vi "Sub UI Update i box.vi"(8 "error in (no error)":errorcluster, 11 "LF2R IDE in":refnum<class "LF2R IDE.lvclass">) -> (0 "error out":errorcluster, 3 "LF2R IDE out":refnum<class "LF2R IDE.lvclass">)   [LabVIEW 2018, in "LF2R IDE.lvlib" / "LF2R IDE.lvclass"]
uses:
  LF2R IDE.lvclass
  LF2R IDE.lvclass/LF2R IDE.ctl
  Image/Image Process.lvclass
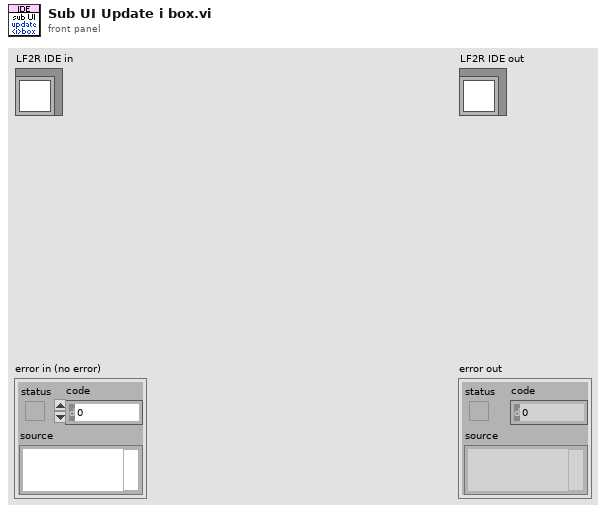
[diagram p1: front panel]
types:
  T1 = typedef "IMAQ Image.ctl" = refnum<image>
  T2 = typedef "Data Parser.lvclass/frame i data.ctl" = cluster{"kind":string, "x":string, "y":string, "w":string, "h":string, "dvx":string, "dvy":string, "dvz":string, "fall":string, "arest":string, "vrest":string, "bdefend":string, "injury":string, "zwidth":string, "effect":string, "catchingact":string, "caughtact":string}
  T3 = cluster{"Fill Color":u32, "Border Color":u32, "Show?":bool}
  T4 = cluster{"x":string, "y":string, "w":string, "h":string}
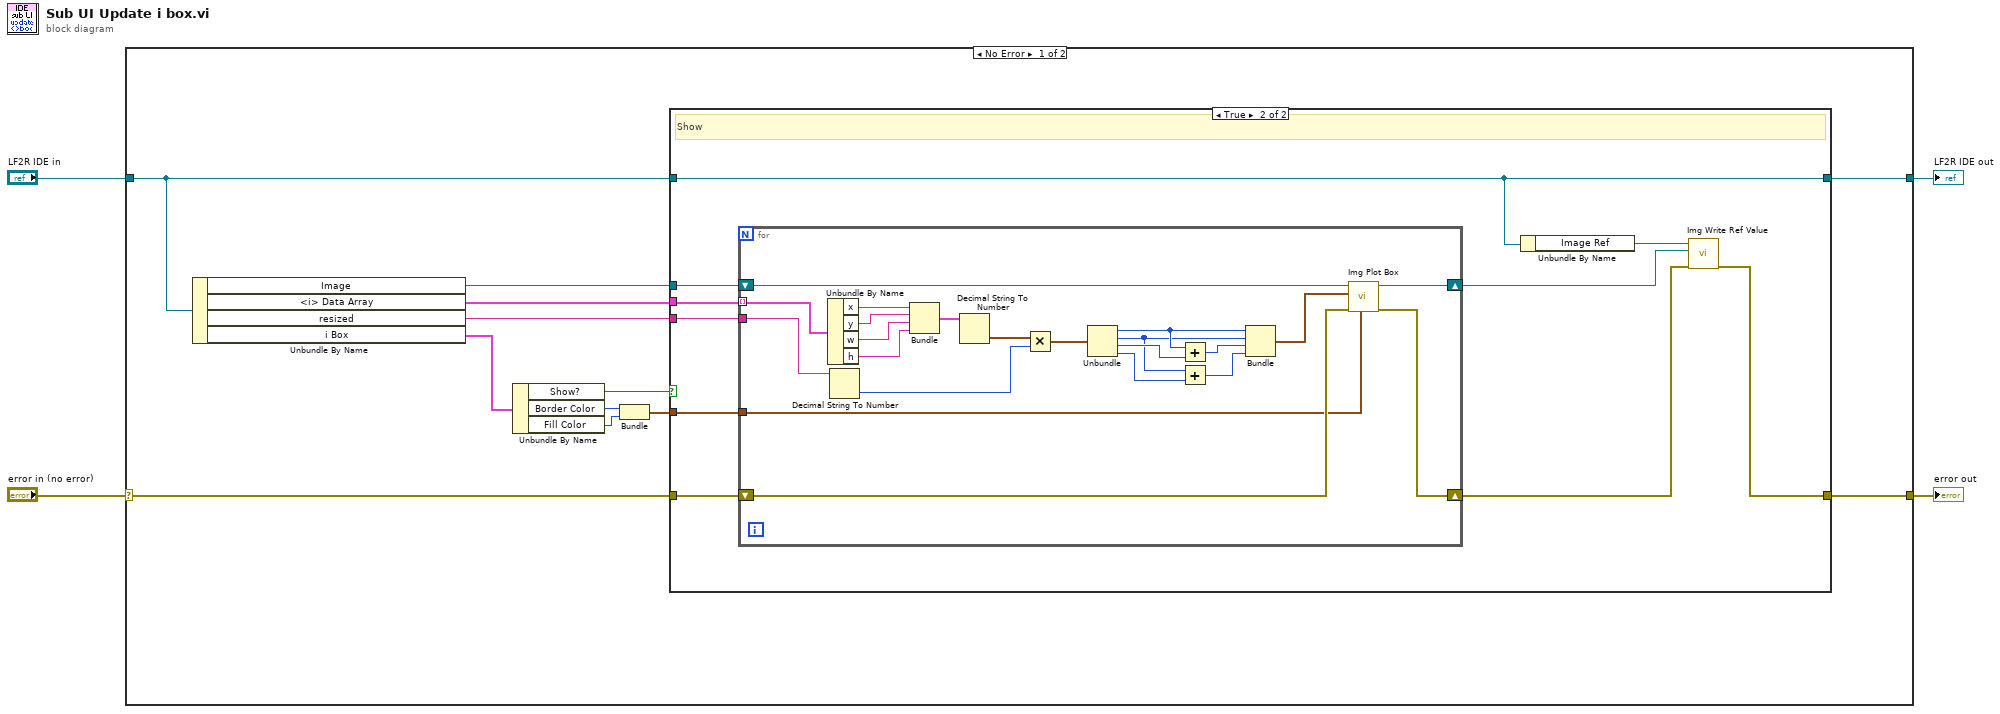
[diagram p0: block diagram]
diagram:
  n1 = case shown="No Error" "error in (no error)" {
    selector: "error in (no error)" -> [w14 w52]
    tunnel: [w12 w52] -> w3
    tunnel: [w9 w51] -> w1
    tunnel: "LF2R IDE in" -> [w13 w51]
    frame No Error {
      n2 = Unbundle By Name(w13) -> ("Image"=w16:T1, "<i> Data Array"=w15:T2[], "resized"=w11:string, "i Box"=w10:T3)
      n3 = Unbundle By Name(w10) -> ("Show?"=w8:bool, "Border Color"=w7:u32, "Fill Color"=w6:u32)
      n4 = Bundle("Border Color"=w7, "Fill Color"=w6) -> (w5:cluster{"Border Color":u32, "Fill Color":u32})  [unwired: 1 in]
      n5 = case shown="True" w8 {
        tunnel: w16 -> [_ w28]
        tunnel: w15 -> [_ w27]
        tunnel: w14 -> [w17 w26]
        tunnel: w13 -> [w18 w20]
        tunnel: [w17 w22] -> w12
        tunnel: w11 -> [_ w21]
        tunnel: [w18 w20] -> w9
        tunnel: w5 -> [_ w19]
        frame False {
          # "Skip"
        }
        frame True {
          # "Show"
          n6 = for {
            tunnel: w27 -> [w49] mode=indexing
            shift-right: [w45] -> w23
            shift-left: w26 -> [w46]
            shift-right: [w44] -> w24
            shift-left: w28 -> [w50]
            tunnel: w21 -> [w31]
            tunnel: w19 -> [w29]
            n7 = Unbundle By Name(w49) -> ("x"=w43:string, "y"=w42:string, "w"=w41:string, "h"=w40:string)
            n8 = Decimal String To Number(string=w31) -> (number=w30:i32)  [unwired: 2 in, 1 out]
            n9 = Bundle("x"=w43, "y"=w42, "w"=w41, "h"=w40) -> (w39:T4)  [unwired: 1 in]
            n10 = Decimal String To Number(string=w39) -> (number=w33:cluster{"x":i32, "y":i32, "w":i32, "h":i32})  [unwired: 2 in, 1 out]
            n11 = Multiply(x=w33, y=w30) -> (x*y=w32:cluster{"x":i32, "y":i32, "w":i32, "h":i32})
            n12 = Unbundle(w32) -> ("x"=w38:i32, "y"=w36:i32, "w"=w37:i32, "h"=w35:i32)
            n13 = Add(x=w38, y=w37) -> (x+y=w48:i32)
            n14 = Add(x=w36, y=w35) -> (x+y=w47:i32)
            n15 = Bundle("x"=w38, "y"=w36, w48, w47) -> (w34:cluster{"x":i32, "y":i32, i32, i32})  [unwired: 1 in]
            n16 = call "Img Plot Box.vi"("Color"=w29, "error in (no error)"=w46, "Rectangle"=w34, "Image in"=w50) -> ("error out"=w45:errorcluster, "Image Out"=w44:T1)  [unwired: 6 in]
          }
          n17 = Unbundle By Name(w20) -> ("Image Ref"=w25:refnum<vi>)
          n18 = call "Img Write Ref Value.vi"("error in (no error)"=w23, "Image"=w24, "Image Ref"=w25) -> ("error out"=w22:errorcluster)  [unwired: 8 in]
        }
      }
    }
    frame Error {
    }
  }
  "error out" <- w3
  "LF2R IDE out" <- w1
